vi "Lex.vi"(8 "Error In":errorcluster, 11 "Compiler In":refnum<class "Compiler.lvclass">) -> (0 "Error Out":errorcluster, 2 "Tokens":refnum<class "Token.lvclass">[](array[class]), 3 "Compiler Out":refnum<class "Compiler.lvclass">)   [LabVIEW 2018, in "Toolkit.lvlib" / "Compiler.lvclass"]
uses:
  Compiler.lvclass
  Tokens/Token/Token.lvclass
  Compiler.lvclass/Compiler.ctl
  Lexer/Lexer.lvclass
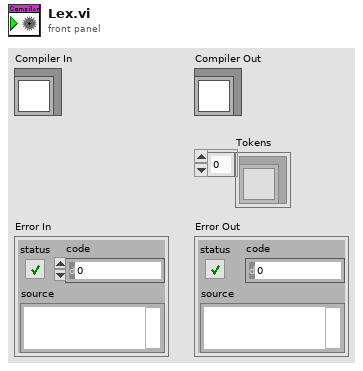
[diagram p1: front panel]
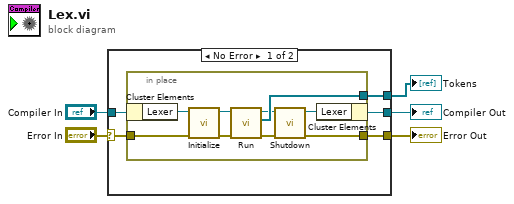
[diagram p0: block diagram]
diagram:
  n1 = case shown="No Error" "Error In" {
    selector: "Error In" -> [w6 w20]
    tunnel: [w10 w20] -> w5
    tunnel: [w9 _] -> w4
    tunnel: [w8 w21] -> w3
    tunnel: "Compiler In" -> [w7 w21]
    frame No Error {
      n2 = in-place {
        in-place-border: [w19] -> w9
        in-place-border: [w13] -> w10
        in-place-border: w6 -> [w11]
        n3 = in-place-cluster #1(w7) -> ("Lexer"=w12:refnum<class "Lexer.lvclass">)
        n4 = call-dynamic "Initialize.vi"("Error In"=w11, "Lexer In"=w12) -> ("Error Out"=w15:errorcluster, "Lexer Out"=w18:refnum<class "Lexer.lvclass">)  [unwired: 8 in]
        n5 = call-dynamic "Run.vi"("Error In"=w15, "Lexer In"=w18) -> ("Error Out"=w14:errorcluster, "Tokens"=w19:refnum<class "Token.lvclass">[], "Lexer Out"=w17:refnum<class "Lexer.lvclass">)  [unwired: 7 in]
        n6 = call-dynamic "Shutdown.vi"("Error In"=w14, "Lexer In"=w17) -> ("Error Out"=w13:errorcluster, "Lexer Out"=w16:refnum<class "Lexer.lvclass">)  [unwired: 8 in]
        n7 = in-place-cluster #1("Lexer"=w16) -> (w8:refnum<class "Compiler.lvclass">)
      }
    }
    frame Error {
    }
  }
  "Error Out" <- w5
  "Tokens" <- w4
  "Compiler Out" <- w3
